vi "Configure Power.vi"(0 "VISA resource name":refnum<visa-resource-name>, 1 "Channel (1)":i32=1, 2 "Port (1)":i32=1, 3 "Port Coupling (T: On)":bool=TRUE, 5 "Power Level (0.0)":dbl format="%^.2g", 11 "error in (no error)":errorcluster, 12 "Power Slope (F: Off)":bool, 13 "Power Slope Coefficient (0.0)":dbl format="%^.2g") -> (4 "VISA resource name out":refnum<visa-resource-name>, 15 "error out":errorcluster)   [LabVIEW 2012, in "Tektronix TTR500 Series.lvlib"]
doc: "This VI configures power settings."
uses:
  <instrlib>/Tektronix TTR500 Series/Tektronix TTR500 Series.lvlib
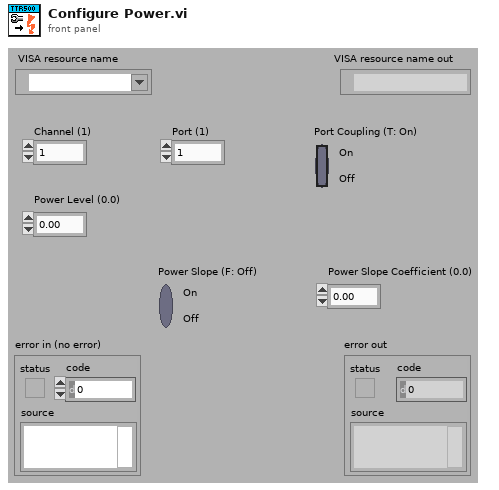
[diagram p1: front panel]
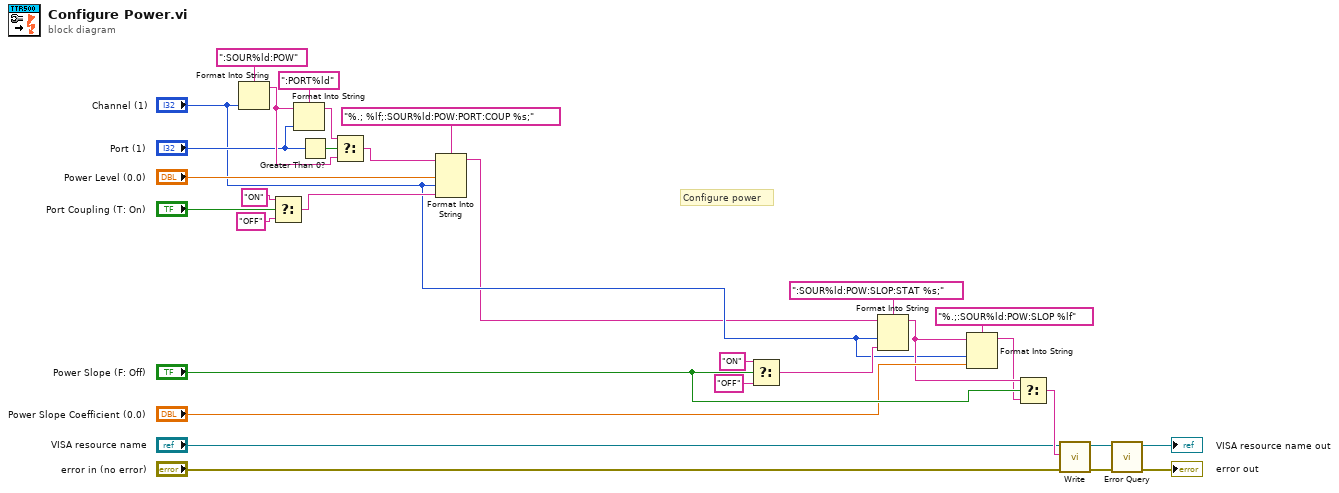
[diagram p0: block diagram]
diagram:
  # "Configure power"
  n1 = Format Into String(format string=":SOUR%ld:POW", "Channel (1)") -> (resulting string=w27:string)  [unwired: 2 in, 1 out]
  n2 = Select(t="ON", s="Port Coupling (T: On)", f="OFF") -> (s? t:f=w19:string)
  n3 = Format Into String(format string=":PORT%ld", initial string=w27, "Port (1)") -> (resulting string=w26:string)  [unwired: 1 in, 1 out]
  n4 = Greater Than 0?(x="Port (1)") -> (x > 0?=w28:bool)
  n5 = Select(t=w26, s=w28, f=w27) -> (s? t:f=w24:string)
  n6 = Format Into String(format string="%.; %lf;:SOUR%ld:POW:PORT:COUP %s;", initial string=w24, "Power Level (0.0)", "Channel (1)", w19) -> (resulting string=w3:string)  [unwired: 1 in, 1 out]
  n7 = Select(t="ON", s="Power Slope (F: Off)", f="OFF") -> (s? t:f=w15:string)
  n8 = Format Into String(format string=":SOUR%ld:POW:SLOP:STAT %s;", initial string=w3, "Channel (1)", w15) -> (resulting string=w11:string)  [unwired: 1 in, 1 out]
  n9 = Format Into String(format string="%.;:SOUR%ld:POW:SLOP %lf", initial string=w11, "Channel (1)", "Power Slope Coefficient (0.0)") -> (resulting string=w10:string)  [unwired: 1 in, 1 out]
  n10 = Select(t=w11, s="Power Slope (F: Off)", f=w10) -> (s? t:f=w9:string)
  n11 = call <instrlib>:"Write.vi"("error in (no error)"="error in (no error)", "String ()"=w9, "VISA resource name"="VISA resource name") -> ("error out"=w7:errorcluster, "VISA resource name out"=w8:refnum<visa-resource-name>)  [unwired: 6 in, 1 out]
  n12 = call <instrlib>:"Error Query.vi"("error in (no error)"=w7, "VISA resource name"=w8) -> ("error out"=→"error out":errorcluster, "VISA resource name out"=→"VISA resource name out":refnum<visa-resource-name>)  [unwired: 6 in, 2 out]
